vi "GFITS_FindKeywordFromArray.vi"(10 "Keyword":string, 11 "Keywords":string[][][](array[string])) -> (1 "found":bool, 2 "values":string[][](array[string]), 3 "indexes":i16[](array[numeric]))   [LabVIEW 2016]
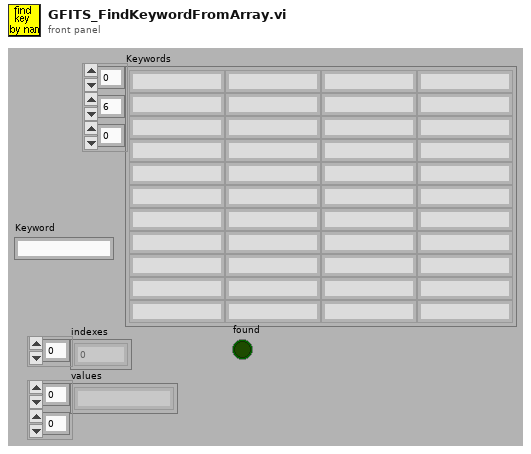
[diagram p1: front panel]
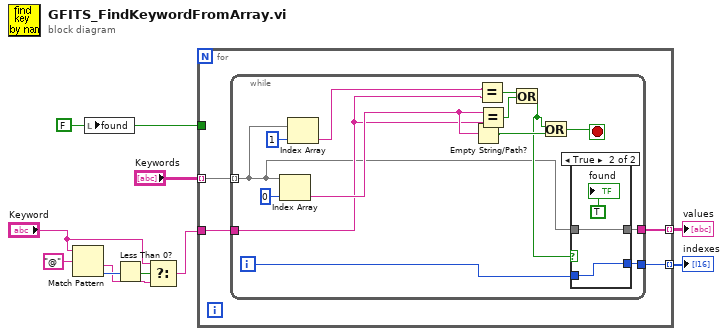
[diagram p0: block diagram]
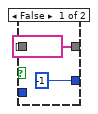
[diagram p2: hidden frame]
diagram:
  w7 = FALSE ("found")
  n1 = Match Pattern(string="Keyword", regular expression="@") -> (after substring=w2:string, offset past match=w5:i32)  [unwired: 3 out]
  n2 = local write "found"(w7) -> ()
  n3 = Less Than 0?(x=w5) -> (x < 0?=w3:bool)
  n4 = Select(t="Keyword", s=w3, f=w2) -> (s? t:f=w1:string)
  n5 = for {
    tunnel: "Keywords" -> [w14] mode=indexing
    tunnel: w1 -> [w13]
    tunnel: [w12] -> w9 mode=indexing
    tunnel: [w11] -> w8 mode=indexing
    tunnel: w7 -> [_]
    n6 = while {
      tunnel: [w22] -> w11
      tunnel: [w23] -> w12
      tunnel: w13 -> [w19]
      tunnel: w14 -> [w18] mode=indexing
      i -> [w24]
      stop <- w28 stop-if-true
      n7 = Index Array(array=w18, index=0 ("Index")) -> (element=w26:string)
      n8 = Index Array(array=w18, index=1) -> (element=w16:string)
      n9 = Empty String/Path?(string/path=w26) -> (empty?=w25:bool)
      n10 = Equal?(x=w16, y=w19) -> (x = y?=w15:bool)
      n11 = Equal?(x=w26, y=w19) -> (x = y?=w21:bool)
      n12 = Or(x=w15, y=w21) -> (x .or. y?=w20:bool)
      n13 = Or(x=w20, y=w25) -> (x .or. y?=w28:bool)
      n14 = case shown="True" w20 {
        tunnel: w24 -> [_ w33]
        tunnel: [-1 w33] -> w23
        tunnel: w18 -> [_ w32]
        tunnel: [string[] [] ("Keywords") w32] -> w22
        frame False {
        }
        frame True {
          "found" <- TRUE ("found")
        }
      }
    }
  }
  "indexes" <- w9
  "values" <- w8
